vi "Update Columns Ctl OoC.vi"(4 "Project Ref":refnum<vi>, 5 "Type Path Map":map{path, path}(c390), 6 "Names":string[](array[string]), 7 "Entity Paths":T1, 8 "error in (no error)":errorcluster, 11 "Updated Definition":refnum<class "Type.lvclass">[](array[class])) -> (0 "error":errorcluster)   [LabVIEW 2020, in "Conditum-Tools.lvlib" / "Entity Editor.lvclass"]
uses:
  Entity Editor.lvclass
  Conditum-Clone/Columns/Type/Type.lvclass
  Entity Paths.ctl
  <vilib>/Utility/miscctls.llb/LVPointTypeDef.ctl
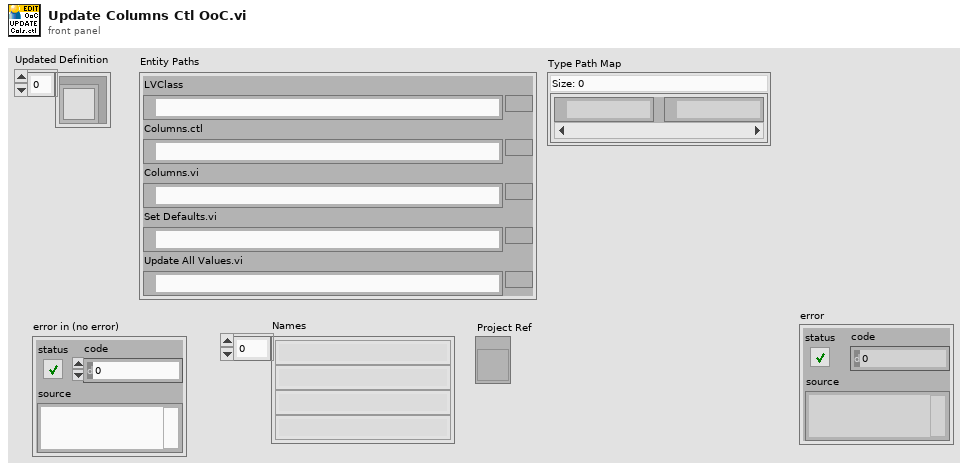
[diagram p1: front panel]
types:
  T1 = typedef "Conditum-Tools.lvlib/Entity Editor.lvclass/Entity Paths.ctl" = cluster{"LVClass":path, "Columns.ctl":path, "Columns.vi":path, "Set Defaults.vi":path, "Update All Values.vi":path}
  T2 = enum32{"invalid lock state", "Not Locked", "Locked (No Password)", "Password-protected"}
  T3 = typedef "LVPointTypeDef.ctl" = cluster{"Horizontal":i16, "Vertical":i16}
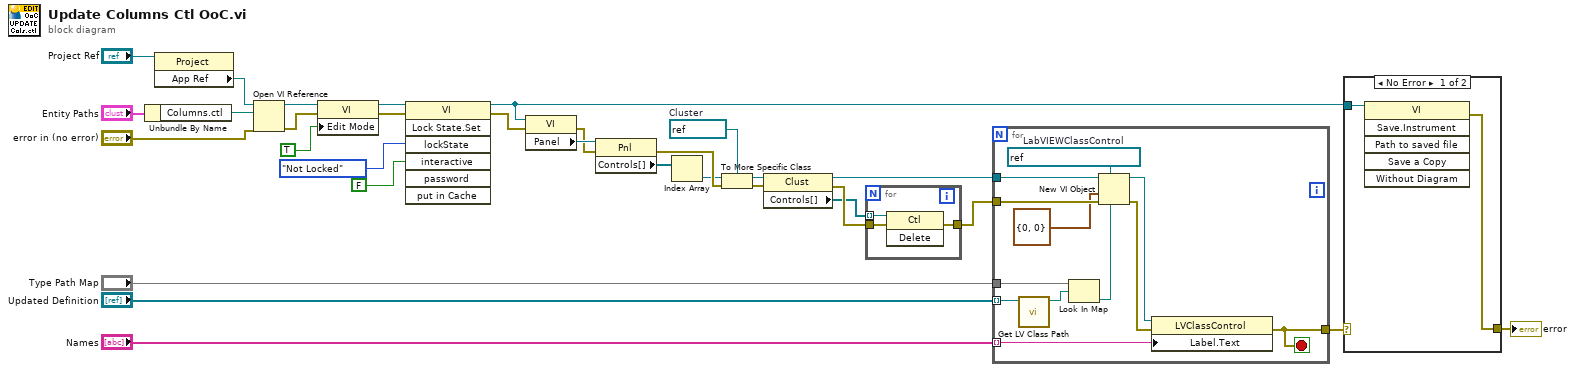
[diagram p0: block diagram]
diagram:
  w24 = refnum<vi> refnum  # Cluster
  n1 = Unbundle By Name("Entity Paths") -> ("Columns.ctl"=w28:path)
  n2 = property class="Project"(reference="Project Ref") -> ("App Ref"=w2:refnum<vi>)  [unwired: 1 in, 2 out]
  n3 = Open VI Reference(application reference (local)=w2, vi path=w28, error in (no error)="error in (no error)") -> (vi reference=w12:refnum<vi>, error out=w11:errorcluster)  [unwired: 3 in]
  n4 = property class="VI"(reference=w12, error in=w11, "Edit Mode"=TRUE ("Edit Mode On Open")) -> (reference out=w7:refnum<vi>, error out=w6:errorcluster)
  n5 = invoke class="VI" method="Lock State.Set"(reference=w7, error in=w6, "lockState"=T2."Not Locked" ("Lock State"), "interactive"=FALSE ("Interactive")) -> (reference out=w5:refnum<vi>, error out=w4:errorcluster)  [unwired: 3 in, 5 out]
  n6 = property class="VI"(reference=w5, error in=w4) -> (error out=w21:errorcluster, "Panel"=w27:refnum<vi>)  [unwired: 1 out]
  n7 = property class="Pnl"(reference=w27, error in=w21) -> (error out=w31:errorcluster, "Controls[]"=w26:refnum<vi>[])  [unwired: 1 out]
  n8 = Index Array(array=w26) -> (element=w25:refnum<vi>)  [unwired: 1 in]
  n9 = To More Specific Class(target class=w24, reference=w25, error in=w31) -> (specific class reference=w23:refnum<vi>, error out=w20:errorcluster)
  n10 = property class="Clust"(reference=w23, error in=w20) -> (reference out=w19:refnum<vi>, error out=w30:errorcluster, "Controls[]"=w22:refnum<vi>[])
  n11 = for {
    tunnel: w22 -> [w34] mode=indexing
    tunnel: [w33] -> w18
    tunnel: w30 -> [w32]
    n12 = invoke class="Ctl" method="Delete"(reference=w34, error in=w32) -> (error out=w33:errorcluster)  [unwired: 1 in, 2 out]
  }
  n13 = for {
    tunnel: w18 -> [w45]
    tunnel: "Updated Definition" -> [w43] mode=indexing
    tunnel: "Names" -> [w40] mode=indexing
    tunnel: w19 -> [w46]
    tunnel: [w38] -> w15
    tunnel: "Type Path Map" -> [w37]
    stop <- w38 stop-if-true
    w44 = refnum<vi> refnum  # LabVIEWClassControl
    n14 = call <vilib>:"Get LV Class Path.vi"("object"=w43) -> ("class path"=w36:path)  [unwired: 9 in, 1 out]
    n15 = Look In Map(map=w37, key=w36) -> (value=w35:path)  [unwired: 1 in, 1 out]
    n16 = New VI Object(vi object class=w44, owner refnum=w46, position/next to=T3 {"Horizontal"=0, "Vertical"=0} ("location"), 6:w35, 8:w45) -> (object refnum=w41:refnum<vi>, 0:w39:errorcluster)  [unwired: 3 in]
    n17 = property class="LVClassControl"(reference=w41, error in=w39, "Label.Text"=w40) -> (error out=w38:errorcluster)  [unwired: 1 out]
  }
  n18 = case shown="No Error" w15 {
    selector: w15 -> [_ w49]
    tunnel: w5 -> [w48 _]
    tunnel: [w47 w49] -> w14
    frame No Error {
      n19 = invoke class="VI" method="Save.Instrument"(reference=w48) -> (error out=w47:errorcluster)  [unwired: 5 in, 5 out]
    }
    frame Error {
    }
  }
  "error" <- w14
